vi "Get Fingers Position.vi"(8 "error in (no error)":errorcluster, 11 "MF3 in":refnum<class "MF3.lvclass">) -> (0 "error out":errorcluster, 1 "joint angles":dbl[](array[numeric]), 2 "Thumb position":dbl[](array[numeric]), 3 "MF3 out":refnum<class "MF3.lvclass">)   [LabVIEW 2011, in "MF3.lvclass"]
uses:
  MF3.lvclass
  Controls/Motor Names.ctl
  MF3.lvclass/MF3.ctl
  Finger/Finger.lvclass
  <vilib>/robotics/Kinematics/NI_Kinematics.lvlib
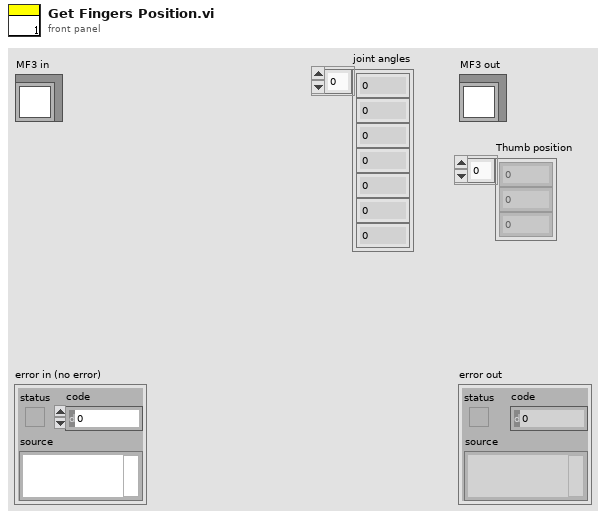
[diagram p1: front panel]
types:
  T1 = typedef "Motor Names.ctl" = enum16{"Thumb1", "Thumb2", "Thumb3", "Index1", "Index2", "Index3", "Redundant", "Middle1", "Middle2", "Middle3"}
  T2 = typedef "NI_Matrix.lvlib/RealMatrix.ctl" = dbl[][]
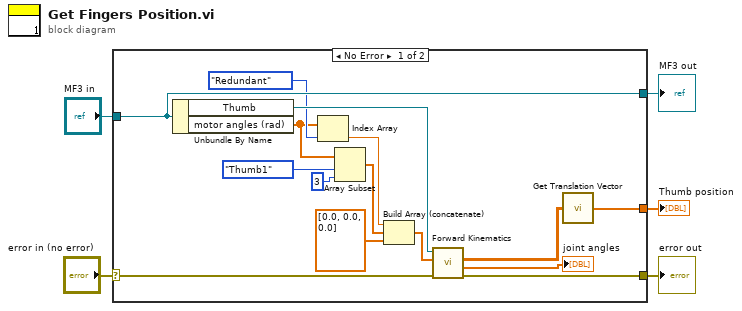
[diagram p0: block diagram]
diagram:
  n1 = case shown="No Error" "error in (no error)" {
    selector: "error in (no error)" -> [w18 w22]
    tunnel: [w17 w22] -> w4
    tunnel: [w20 w21] -> w2
    tunnel: "MF3 in" -> [w20 w21]
    tunnel: [w15 _] -> w1
    frame No Error {
      n2 = Unbundle By Name(w20) -> ("Thumb"=w19:refnum<class "Finger.lvclass">, "motor angles (rad)"=w8:dbl[])
      n3 = Index Array(array=w8, index=Motor_Names."Redundant" ("Motor Names")) -> (element=w7:dbl)
      n4 = Array Subset(array=w8, index=Motor_Names."Thumb1" ("Motor Names"), length=3) -> (w9:dbl[])
      n5 = Build Array (concatenate)(w7, w9, dbl[] [0.0, 0.0, 0.0] ("subarray")) -> (w13:dbl[])
      n6 = call "Forward Kinematics.vi"("error in (no error)"=w18, "motor angles"=w13, "Finger in"=w19) -> ("error out"=w17:errorcluster, "joint angles"=→"joint angles":dbl[], "T"=w16:T2)  [unwired: 5 in, 1 out]
      n7 = call <vilib>:"Get Translation Vector.vi"("transform"=w16) -> ("translation vector"=w15:dbl[])
    }
    frame Error {
    }
  }
  "error out" <- w4
  "MF3 out" <- w2
  "Thumb position" <- w1
